vi "TEST X Listbox-Solution.vi"() -> ()   [LabVIEW 2011]
doc: "This is the solution for the Test VI.\n\nAAL 9/09"
uses:
  X Listbox-Solution.xctl
panel:
  in  "X Listbox":string(xcontrol)
  out "Deleted Item":string
  out "Invalid Item?":bool
  in  "Delete All":bool
  in  "Item Name":string
  in  "Add Item":bool
  in  "Delete Item":bool
  in  "Delete Item":string
  in  "Exit":bool
  out "X Control Output":string
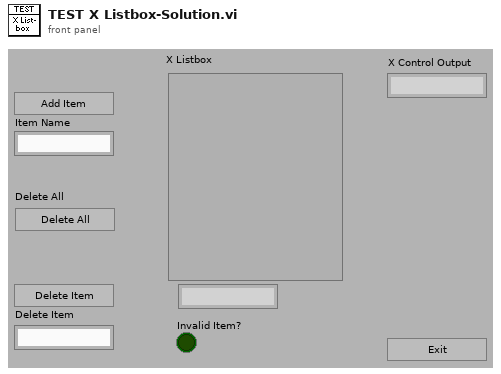
[diagram p1: front panel]
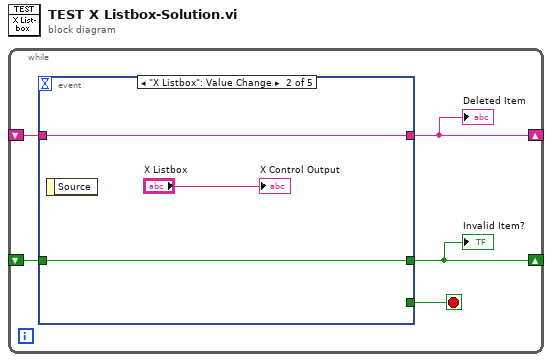
[diagram p0: block diagram]
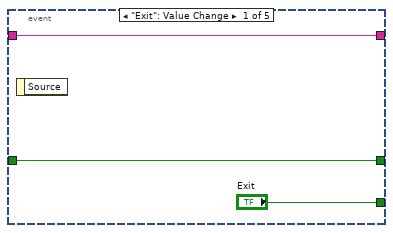
[diagram p2: hidden frame]
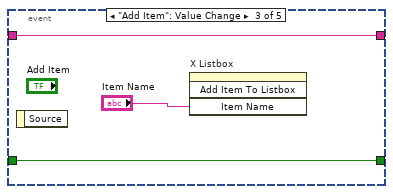
[diagram p3: hidden frame]
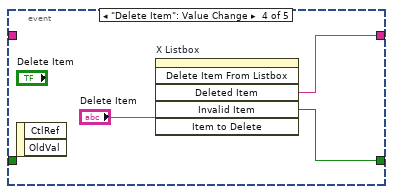
[diagram p4: hidden frame]
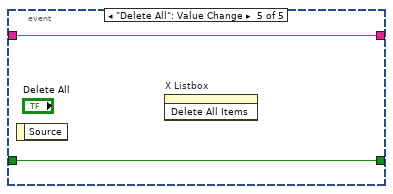
[diagram p5: hidden frame]
diagram:
  n1 = while {
    shift-right: [w4] -> _
    shift-left: _ -> [w3]
    shift-right: [w2] -> _
    shift-left: _ -> [w1]
    stop <- w5 stop-if-true
    n2 = event shown="[1] \"X Listbox\": Value Change" {
      selector: _ -> [_ _ _ _ _]
      dyn-events: _ -> [_ _ _ _ _]
      timeout: _ -> [_ _ _ _ _]
      tunnel: ["Exit" _ _ _ _] -> w5
      tunnel: [w6 w9 w12 w16 w18] -> w2
      tunnel: [w7 w10 w13 w15 w19] -> w4
      tunnel: w3 -> [w7 w10 w13 _ w19]
      tunnel: w1 -> [w6 w9 w12 _ w18]
      event "Exit": Value Change {
        n3 = event-data() -> ()  [unwired: 2 out]
      }
      event "X Listbox": Value Change {
        n4 = event-data() -> ()  [unwired: 2 out]
        "X Control Output" <- "X Listbox"
      }
      event "Add Item": Value Change {
        n5 = event-data() -> ()  [unwired: 2 out]
        n6 = invoke on="X Listbox" class="X Listbox-Solution (strict)" method="Add Item To Listbox"("Item Name"="Item Name") -> ()  [unwired: 3 in, 4 out]
      }
      event "Delete Item": Value Change {
        n7 = event-data() -> ()  [unwired: 3 out]
        n8 = invoke on="X Listbox" class="X Listbox-Solution (strict)" method="Delete Item From Listbox"("Item to Delete"="Delete Item") -> ("Deleted Item"=w15:string, "Invalid Item"=w16:bool)  [unwired: 5 in, 4 out]
      }
      event "Delete All": Value Change {
        n9 = event-data() -> ()  [unwired: 2 out]
        n10 = invoke on="X Listbox" class="X Listbox-Solution (strict)" method="Delete All Items"() -> ()  [unwired: 3 in, 3 out]
      }
    }
    "Invalid Item?" <- w2
    "Deleted Item" <- w4
  }
